vi "fetch_scan_head.vi"(8 "error in (no error)":errorcluster) -> (0 "error out":errorcluster, 3 "GenericScanHead out":refnum<class "GenericScanHead.lvclass">)   [LabVIEW 2010]
uses:
  class_data.vi
  GenericScanHead.lvclass
  common/classes/ErrorController/ErrorController/ErrorController.lvclass
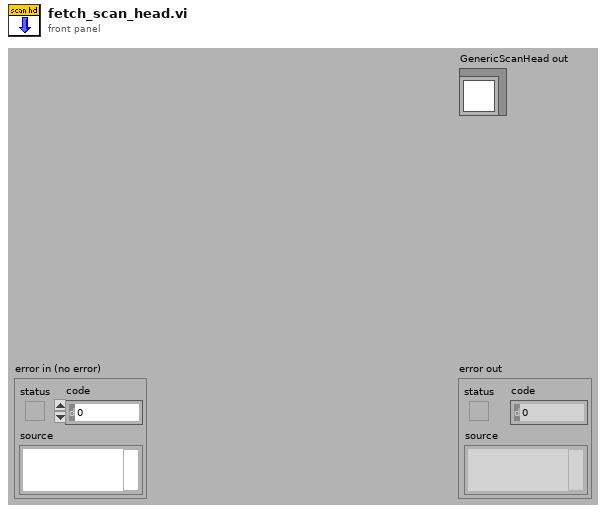
[diagram p1: front panel]
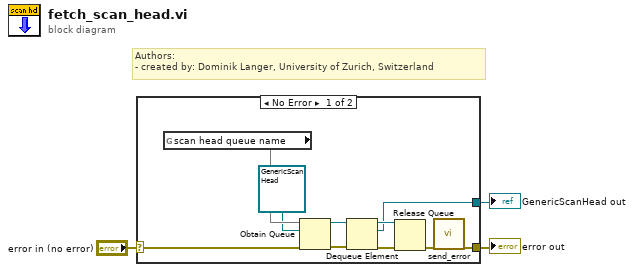
[diagram p0: block diagram]
diagram:
  # "Authors: \n- created by: Dominik Langer, University of Zurich, Switzerland"
  n1 = case shown="No Error" "error in (no error)" {
    selector: "error in (no error)" -> [w11 w14]
    tunnel: [w4 w14] -> w2
    tunnel: [w6 _] -> w1
    frame No Error {
      n2 = global read "class_data.vi" "scan head queue name"() -> (w13)
      n3 = Obtain Queue(name (unnamed)=w13, element data type=refnum<class "GenericScanHead.lvclass"> refnum ("GenericScanHead.lvclass"), error in (no error)=w11) -> (queue out=w9:refnum<queue>, error out=w12:errorcluster)  [unwired: 2 in, 1 out]
      n4 = Dequeue Element(queue=w9, error in (no error)=w12) -> (queue out=w7:refnum<queue>, element=w6:refnum<class "GenericScanHead.lvclass">, error out=w8:errorcluster)  [unwired: 2 out]
      n5 = Release Queue(queue=w7, error in (no error)=w8) -> (error out=w5:errorcluster)  [unwired: 3 out]
      n6 = call "send_error.vi"("error in (no error)"=w5) -> ("error out"=w4:errorcluster)  [unwired: 10 in]
    }
    frame Error {
    }
  }
  "error out" <- w2
  "GenericScanHead out" <- w1
